vi "Modbus Send Parameters FVIR.vi"(8 "error in (no error)":errorcluster, 10 "Array":i32[](array[numeric]), 11 "Modbus Master in":refnum<class "Modbus Master.lvclass">) -> (0 "error out":errorcluster, 3 "Modbus Master out":refnum<class "Modbus Master.lvclass">)   [LabVIEW 2020, in "Modbus.lvlib"]
uses:
  Modbus.lvlib
  <vilib>/NI/Modbus Library/API/Master/Modbus Master.lvclass
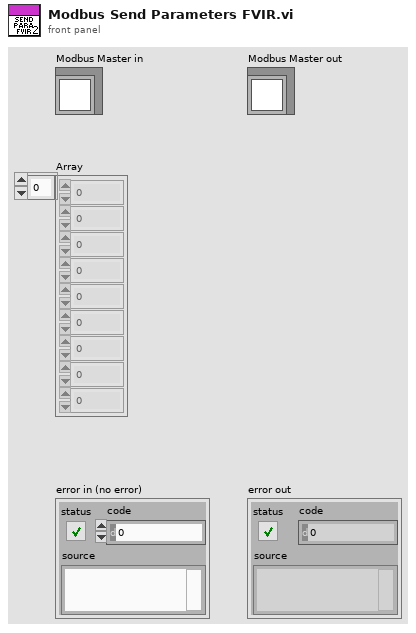
[diagram p1: front panel]
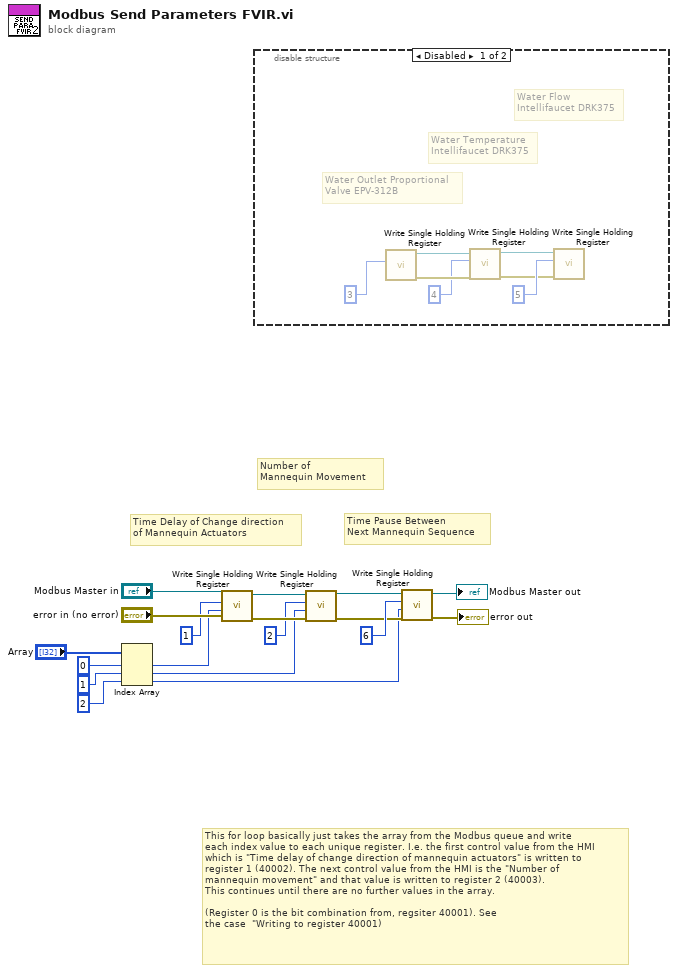
[diagram p0: block diagram]
diagram:
  # "This for loop basically just takes the array from the Modbus queue and write\neach index value to each unique register. I.e. the first control value from the HMI\nwhich is \"Time delay of change direction of mannequin actuators\" is written to \nregister 1 (40002). The next control value from the HMI is the \"Number of\nmannequin movement\" and that value is written to register 2 (40003). \nThis continues until there are no further values in the array.\n\n(Register 0 is the bit combination from, regsiter 40001). See\nthe case  \"Writing to register 40001)"
  # "Time Pause Between\nNext Mannequin Sequence"
  # "Number of\nMannequin Movement"
  # "Time Delay of Change direction\nof Mannequin Actuators"
  n1 = Index Array(array="Array", index #1=0 ("index"), index #2=1 ("index"), index #3=2 ("index")) -> (element #1=w9:i32, element #2=w8:i32, element #3=w1:i32)
  n2 = call-dynamic "Write Single Holding Register.vi"("error in"="error in (no error)", "register to write"=w9, "address"=u16 1, "Modbus master in"="Modbus Master in") -> ("error out"=w13:errorcluster, "Modbus master out"=w18:refnum<class "Modbus Master.lvclass">)  [unwired: 6 in]
  n3 = disable-structure shown="Disabled" {
    frame Disabled {
      # "Water Flow\nIntellifaucet DRK375"
      # "Water Temperature\nIntellifaucet DRK375"
      # "Water Outlet Proportional\nValve EPV-312B"
      n4 = call-dynamic "Write Single Holding Register.vi"("address"=u16 3) -> ("error out"=w24:errorcluster, "Modbus master out"=w25:refnum<class "Modbus Master.lvclass">)  [unwired: 9 in]
      n5 = call-dynamic "Write Single Holding Register.vi"("error in"=w24, "address"=u16 4, "Modbus master in"=w25) -> ("error out"=w20:errorcluster, "Modbus master out"=w19:refnum<class "Modbus Master.lvclass">)  [unwired: 7 in]
      n6 = call-dynamic "Write Single Holding Register.vi"("error in"=w20, "address"=u16 5, "Modbus master in"=w19) -> ()  [unwired: 7 in, 2 out]
    }
    frame Enabled {
    }
  }
  n7 = call-dynamic "Write Single Holding Register.vi"("error in"=w13, "register to write"=w8, "address"=u16 2, "Modbus master in"=w18) -> ("error out"=w4:errorcluster, "Modbus master out"=w3:refnum<class "Modbus Master.lvclass">)  [unwired: 6 in]
  n8 = call-dynamic "Write Single Holding Register.vi"("error in"=w4, "register to write"=w1, "address"=u16 6, "Modbus master in"=w3) -> ("error out"=→"error out":errorcluster, "Modbus master out"=→"Modbus Master out":refnum<class "Modbus Master.lvclass">)  [unwired: 6 in]
